vi "Get UI Reference.vi"(8 "error in (no error)":errorcluster, 10 "VI Type":refnum<vi>, 11 "Sequencer in":refnum<class "Sequencer.lvclass">) -> (0 "error out":errorcluster, 3 "VI Reference":refnum<vi>)   [LabVIEW 2020]
uses:
  Sequencer.lvclass
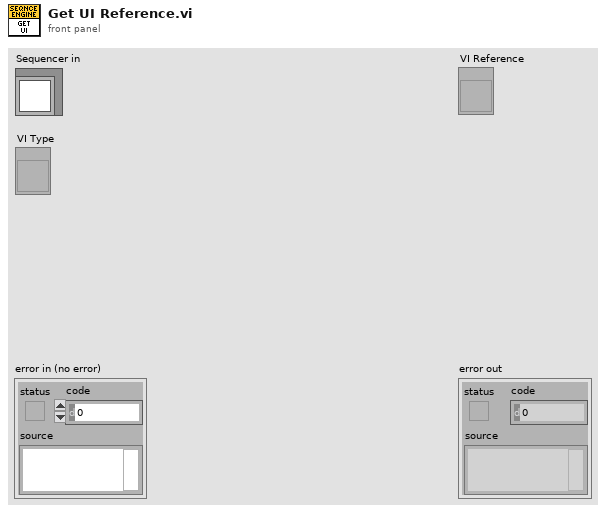
[diagram p1: front panel]
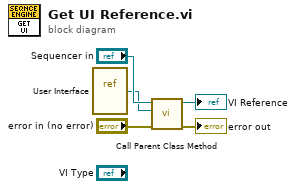
[diagram p0: block diagram]
diagram:
  n1 = vi-ref "User Interface.vi"() -> (w1:refnum<vi>)
  n2 = call-parent "Call Parent Class Method"("error in (no error)"="error in (no error)", "VI Type"=w1, "Service in"="Sequencer in") -> ("error out"=→"error out":errorcluster, "VI Reference"=→"VI Reference":refnum<vi>)  [unwired: 7 in]
